vi "Control - Spark.vi"(8 "Control Inputs":T1={"Engine Speed [RPM]"=0.0, "Engine Status"=enum."STALLED", "Load Control \nMode"=enum."Max Speed Governor", "dt(s)"=0.0, "Number of Cylinders"=0, "Engine Displacement [cc]"=0.0, "StoichAFR"=0.0, "Q.LHV Fuel [kJ/kg]"=0.0, "BattV PSU [V]"=0.0, "12V PSU [V]"=0.0, "5V PSU [V]"=0.0, "Pedal Position [%]"=0.0, "Oil Pressure [kPa]"=0.0, "Oil Temp [C]"=0.0, "Oil Level [%]"=0.0, "Engine Coolant Temp (ECT) [C]"=0.0, "Engine Coolant Pressure [kPa]"=0.0, "Rail Pressure [bar]"=0.0, "Fuel Pressure [kPa]"=0.0, "Fuel Temp [C]"=0.0, "Vacuum Pressure [kPa]"=0.0, "Throttle Position [%]"=0.0, "Cam1 Advance [CAD]"=0.0, "Cam2 Advance [CAD]"=0.0, "Cam3 Advance [CAD]"=0.0, "Cam4 Advance [CAD]"=0.0, "CA50 Control Output [CAD]"=[], "CA50 Control Output Valid"=[], "Intake Air Temp (IAT) [C]"=0.0, "Barometric Air Pressure [kPa]"=0.0, "Intake Air Rel. Humidity [%]"=0.0, "Mass Air Flow (MAF) [kg/hr]"=0.0, "Turbo Inlet Air Pressure [kPa]"=0.0, "Turbo Inlet Air Temp [C]"=0.0, "Turbo Outlet Air Pressure [kPa]"=0.0, "Turbo Outlet Air Temp [C]"=0.0, "CAC Outlet Pressure [kPa]"=0.0, "CAC Outlet Temp [C]"=0.0, "Intake Manifold Pressure (MAP) [kPa]"=0.0, "Intake Manifold Temp (MAT) [C]"=0.0, "Exhaust Manifold Pressure [kPa]"=0.0, "Exhaust Manifold Temp [C]"=0.0, "HighP EGR Cooler Outlet Pressure [kPa]"=0.0, "HighP EGR Cooler Outlet Temp [C]"=0.0, "HighP EGR Differential Pressure [kPa]"=0.0, "HighP EGR Valve Position [%]"=0.0, "Turbo Outlet Exhaust Pressure [kPa]"=0.0, "Turbo Outlet Exhaust Temp [C]"=0.0, "VGT Position 1 [%]"=0.0, "VGT Position 2 [%]"=0.0, "Turbo Speed 1 [RPM]"=0.0, "Turbo Speed 2 [RPM]"=0.0, "LowP EGR Differential Pressure [kPa]"=0.0, "LowP EGR Valve Position [%]"=0.0, "UEGO1Lambda"=0.0, "UEGO1_Hot"=FALSE, "UEGO2Lambda"=0.0, "UEGO2_Hot"=FALSE, "Knock Intensity"=[], "Knock"=[]} {"Knock Intensity" format="%.2f"; "CA50 Control Output [CAD]" format="%.2f"; "Exhaust Manifold Temp [C]" format="%#_6f"; "UEGO2Lambda" format="%.2f"; "Intake Manifold Temp (MAT) [C]" format="%#_6f"; "UEGO1Lambda" format="%.2f"}, 10 "EGR Mass [mg/cyc]":sgl, 11 "MEP Desired [bar]":sgl) -> (1 "Spark Timings Desired [DBTDC]":sgl[](array[numeric]), 3 "Spark Dwells Desired [msec]":sgl[](array[numeric]))   [LabVIEW 2015, in "ECS-RT.lvlib"]
uses:
  ECS-RT.lvlib
  Typedefs/Control Inputs/Control Inputs.ctl
  Typedefs/EPT/Engine Status.ctl
  Typedefs/MISC/Load Control Mode.ctl
  ECS-Shared.lvlib
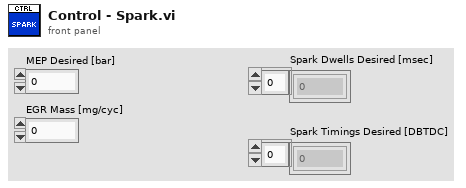
[diagram p1: front panel]
types:
  T1 = typedef "ECS-Shared.lvlib/Control Inputs.ctl" = cluster{"Engine Speed [RPM]":sgl, "Engine Status":T2, "Load Control \nMode":T3, "dt(s)":sgl, "Number of Cylinders":u8, "Engine Displacement [cc]":sgl, "StoichAFR":sgl, "Q.LHV Fuel [kJ/kg]":sgl, "BattV PSU [V]":sgl, "12V PSU [V]":sgl, "5V PSU [V]":sgl, "Pedal Position [%]":sgl, "Oil Pressure [kPa]":sgl, "Oil Temp [C]":sgl, "Oil Level [%]":sgl, "Engine Coolant Temp (ECT) [C]":sgl, "Engine Coolant Pressure [kPa]":sgl, "Rail Pressure [bar]":sgl, "Fuel Pressure [kPa]":sgl, "Fuel Temp [C]":sgl, "Vacuum Pressure [kPa]":sgl, "Throttle Position [%]":sgl, "Cam1 Advance [CAD]":sgl, "Cam2 Advance [CAD]":sgl, "Cam3 Advance [CAD]":sgl, "Cam4 Advance [CAD]":sgl, "CA50 Control Output [CAD]":sgl[], "CA50 Control Output Valid":bool[], "Intake Air Temp (IAT) [C]":sgl, "Barometric Air Pressure [kPa]":sgl, "Intake Air Rel. Humidity [%]":sgl, "Mass Air Flow (MAF) [kg/hr]":sgl, "Turbo Inlet Air Pressure [kPa]":sgl, "Turbo Inlet Air Temp [C]":sgl, "Turbo Outlet Air Pressure [kPa]":sgl, "Turbo Outlet Air Temp [C]":sgl, "CAC Outlet Pressure [kPa]":sgl, "CAC Outlet Temp [C]":sgl, "Intake Manifold Pressure (MAP) [kPa]":sgl, "Intake Manifold Temp (MAT) [C]":sgl, "Exhaust Manifold Pressure [kPa]":sgl, "Exhaust Manifold Temp [C]":sgl, "HighP EGR Cooler Outlet Pressure [kPa]":sgl, "HighP EGR Cooler Outlet Temp [C]":sgl, "HighP EGR Differential Pressure [kPa]":sgl, "HighP EGR Valve Position [%]":sgl, "Turbo Outlet Exhaust Pressure [kPa]":sgl, "Turbo Outlet Exhaust Temp [C]":sgl, "VGT Position 1 [%]":sgl, "VGT Position 2 [%]":sgl, "Turbo Speed 1 [RPM]":sgl, "Turbo Speed 2 [RPM]":sgl, "LowP EGR Differential Pressure [kPa]":sgl, "LowP EGR Valve Position [%]":sgl, "UEGO1Lambda":sgl, "UEGO1_Hot":bool, "UEGO2Lambda":sgl, "UEGO2_Hot":bool, "Knock Intensity":sgl[], "Knock":bool[]}
  T2 = typedef "ECS-Shared.lvlib/Engine Status.ctl" = enum16{"OFF", "STALLED", "CRANKING", "RUNNING", "ACCEL", "DECEL", "SAFE"}
  T3 = typedef "ECS-Shared.lvlib/Load Control Mode.ctl" = enum16{"No Governor", "Min Speed Governor", "Max Speed Governor"}
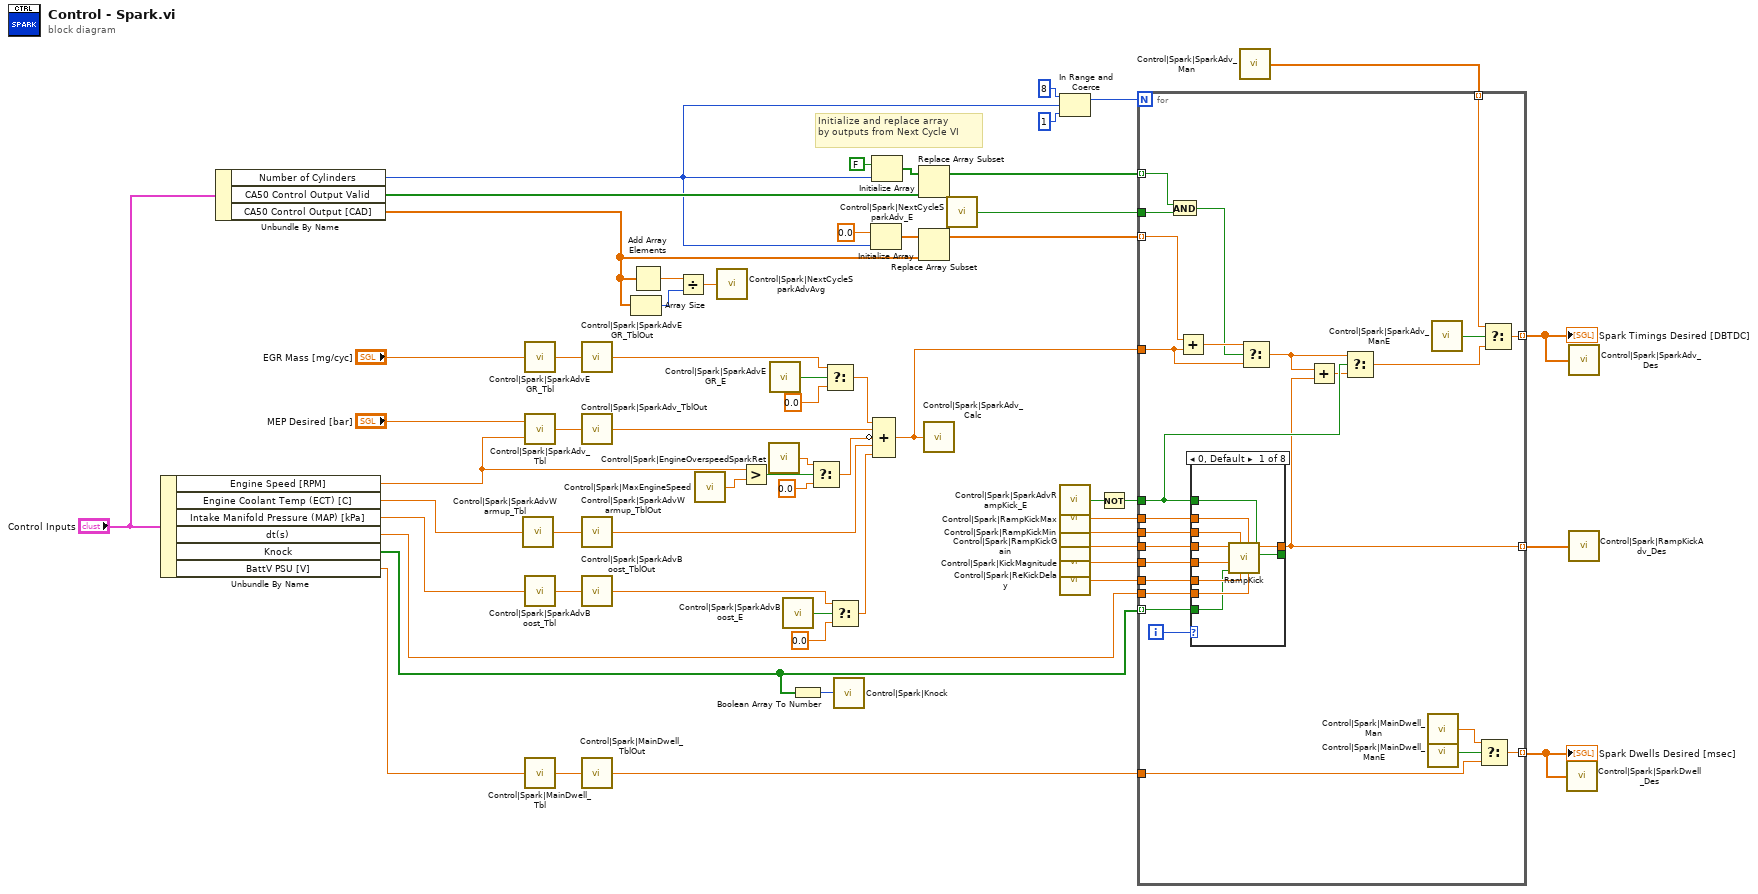
[diagram p0: block diagram]
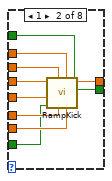
[diagram p2: hidden frame]
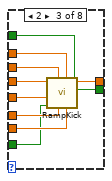
[diagram p3: hidden frame]
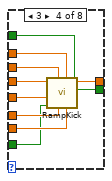
[diagram p4: hidden frame]
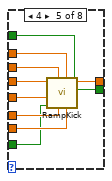
[diagram p5: hidden frame]
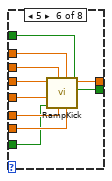
[diagram p6: hidden frame]
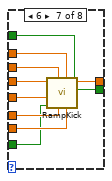
[diagram p7: hidden frame]
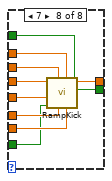
[diagram p8: hidden frame]
diagram:
  # "Initialize and replace array\nby outputs from Next Cycle VI"
  n1 = Unbundle By Name("Control Inputs") -> ("Engine Speed [RPM]"=w26:sgl, "Engine Coolant Temp (ECT) [C]"=w18:sgl, "Intake Manifold Pressure (MAP) [kPa]"=w19:sgl, "dt(s)"=w8:sgl, "Knock"=w7:bool[], "BattV PSU [V]"=w11:sgl)
  n2 = Unbundle By Name("Control Inputs") -> ("Number of Cylinders"=w20:u8, "CA50 Control Output Valid"=w23:bool[], "CA50 Control Output [CAD]"=w22:sgl[])
  n3 = call "Control|Spark|SparkAdvWarmup_Tbl"("X Index"=w18) -> ("Y"=w29:sgl)
  n4 = call "Control|Spark|SparkAdvEGR_Tbl"("X Index"="EGR Mass [mg/cyc]") -> ("Y"=w34:sgl)
  n5 = call "Control|Spark|SparkAdv_Tbl"("Y Index"=w26, "X Index"="MEP Desired [bar]") -> ("Z"=w35:sgl)
  n6 = call "Control|Spark|SparkAdvBoost_Tbl"("X Index"=w19) -> ("Y"=w36:sgl)
  n7 = call "Control|Spark|MainDwell_Tbl"("X Index"=w11) -> ("Y"=w37:sgl)
  n8 = call "Control|Spark|SparkAdvEGR_TblOut"("Value"=w34) -> ()
  n9 = call "Control|Spark|SparkAdv_TblOut"("Value"=w35) -> ()
  n10 = call "Control|Spark|SparkAdvWarmup_TblOut"("Value"=w29) -> ()
  n11 = call "Control|Spark|SparkAdvBoost_TblOut"("Value"=w36) -> ()
  n12 = call "Control|Spark|MainDwell_TblOut"("Value"=w37) -> ()
  n13 = Array Size(array=w22) -> (size(s)=w42:i32)
  n14 = Add Array Elements(numeric array=w22) -> (sum=w43:sgl)
  n15 = Divide(x=w43, y=w42) -> (x/y=w41:sgl)
  n16 = call "Control|Spark|MaxEngineSpeed"() -> ("Value"=w17:sgl)
  n17 = call "Control|Spark|NextCycleSparkAdvAvg"("Value"=w41) -> ()
  n18 = Greater?(x=w26, y=w17) -> (0:w28:bool)
  n19 = call "Control|Spark|EngineOverspeedSparkRet"() -> ("Value"=w25:sgl)
  n20 = call "Control|Spark|SparkAdvEGR_E"() -> ("Value"=w51:bool)
  n21 = call "Control|Spark|SparkAdvBoost_E"() -> ("Value"=w52:bool)
  n22 = Boolean Array To Number(Boolean array=w7) -> (number=w10:u8)
  n23 = Select(t=w25, s=w28, f=sgl 0.0) -> (s? t:f=w27:sgl)
  n24 = Select(t=w34, s=w51, f=sgl 0.0) -> (s? t:f=w48:sgl)
  n25 = Select(t=w36, s=w52, f=sgl 0.0) -> (s? t:f=w30:sgl)
  n26 = call "Control|Spark|Knock"("Value"=w10) -> ()
  n27 = Initialize Array(sgl 0.0, w20) -> (w45:sgl[])
  n28 = Initialize Array(FALSE, w20) -> (w47:bool[])
  n29 = Compound Arithmetic op=ADD(w48, w35, invert w27, w29, w30) -> (w31:sgl)
  n30 = Replace Array Subset(array=w47, new element=w23) -> (w40:bool[])  [unwired: 1 in]
  n31 = Replace Array Subset(array=w45, new element=w22) -> (w39:sgl[])  [unwired: 1 in]
  n32 = call "Control|Spark|SparkAdv_Calc"("Value"=w31) -> ()
  n33 = call "Control|Spark|NextCycleSparkAdv_E"() -> ("Value"=w38:bool)
  n34 = In Range and Coerce(upper limit=u8 8, x=w20, lower limit=u8 1) -> (coerced(x)=w5:u8)  [unwired: 1 out]
  n35 = call "Control|Spark|SparkAdvRampKick_E"() -> ("Value"=w9:bool)
  n36 = call "Control|Spark|RampKickMax"() -> ("Value"=w16:sgl)
  n37 = call "Control|Spark|RampKickMin"() -> ("Value"=w15:sgl)
  n38 = call "Control|Spark|RampKickGain"() -> ("Value"=w14:sgl)
  n39 = call "Control|Spark|KickMagnitude"() -> ("Value"=w13:sgl)
  n40 = call "Control|Spark|ReKickDelay"() -> ("Value"=w12:sgl)
  n41 = Not(x=w9) -> (.not. x?=w6:bool)
  n42 = call "Control|Spark|SparkAdv_Man"() -> ("Value"=w1:sgl[])
  n43 = for {
    N: w5 -> [_]
    tunnel: w31 -> [w74]
    tunnel: w37 -> [w78]
    tunnel: [w77] -> w32 mode=indexing
    tunnel: [w76] -> w33 mode=indexing
    tunnel: w40 -> [w71] mode=indexing
    tunnel: w39 -> [w73] mode=indexing
    tunnel: w38 -> [w70]
    tunnel: w16 -> [w67]
    tunnel: w15 -> [w66]
    tunnel: w14 -> [w65]
    tunnel: w13 -> [w64]
    tunnel: w12 -> [w63]
    tunnel: w8 -> [w62]
    tunnel: w7 -> [w61] mode=indexing
    tunnel: w6 -> [w59]
    tunnel: [w56] -> w2 mode=indexing
    tunnel: w1 -> [w55] mode=indexing
    i -> [w68]
    n44 = And(x=w71, y=w70) -> (x .and. y?=w69:bool)
    n45 = Add(x=w73, y=w74) -> (x+y=w75:sgl)
    n46 = case shown="0, Default" w68 {
      tunnel: w66 -> [w90 w100 w110 w120 w130 w140 w150 w160]
      tunnel: w67 -> [w89 w99 w109 w119 w129 w139 w149 w159]
      tunnel: w65 -> [w88 w98 w108 w118 w128 w138 w148 w158]
      tunnel: w64 -> [w87 w97 w107 w117 w127 w137 w147 w157]
      tunnel: w63 -> [w86 w96 w106 w116 w126 w136 w146 w156]
      tunnel: w62 -> [w85 w95 w105 w115 w125 w135 w145 w155]
      tunnel: w61 -> [w84 w94 w104 w114 w124 w134 w144 w154]
      tunnel: [w83 w93 w103 w113 w123 w133 w143 w153] -> w56
      tunnel: [w82 w92 w102 w112 w122 w132 w142 w152] -> _
      tunnel: w59 -> [w81 w91 w101 w111 w121 w131 w141 w151]
      frame 0, Default {
        n47 = call "RampKick.vi"("Init (F)"=w81, "dt [s]"=w85, "Output Max [unit]"=w89, "Re-Kick Delay [s]"=w86, "Output Min [unit]"=w90, "Kick?"=w84, "Kick Magnitude [unit]"=w87, "Gain [unit/s]"=w88) -> ("Kicked"=w82:bool, "Ramp/Kick Output"=w83:sgl)  [unwired: 2 in]
      }
      frame 1 {
        n48 = call "RampKick.vi"("Init (F)"=w91, "dt [s]"=w95, "Output Max [unit]"=w99, "Re-Kick Delay [s]"=w96, "Output Min [unit]"=w100, "Kick?"=w94, "Kick Magnitude [unit]"=w97, "Gain [unit/s]"=w98) -> ("Kicked"=w92:bool, "Ramp/Kick Output"=w93:sgl)  [unwired: 2 in]
      }
      frame 2 {
        n49 = call "RampKick.vi"("Init (F)"=w101, "dt [s]"=w105, "Output Max [unit]"=w109, "Re-Kick Delay [s]"=w106, "Output Min [unit]"=w110, "Kick?"=w104, "Kick Magnitude [unit]"=w107, "Gain [unit/s]"=w108) -> ("Kicked"=w102:bool, "Ramp/Kick Output"=w103:sgl)  [unwired: 2 in]
      }
      frame 3 {
        n50 = call "RampKick.vi"("Init (F)"=w111, "dt [s]"=w115, "Output Max [unit]"=w119, "Re-Kick Delay [s]"=w116, "Output Min [unit]"=w120, "Kick?"=w114, "Kick Magnitude [unit]"=w117, "Gain [unit/s]"=w118) -> ("Kicked"=w112:bool, "Ramp/Kick Output"=w113:sgl)  [unwired: 2 in]
      }
      frame 4 {
        n51 = call "RampKick.vi"("Init (F)"=w121, "dt [s]"=w125, "Output Max [unit]"=w129, "Re-Kick Delay [s]"=w126, "Output Min [unit]"=w130, "Kick?"=w124, "Kick Magnitude [unit]"=w127, "Gain [unit/s]"=w128) -> ("Kicked"=w122:bool, "Ramp/Kick Output"=w123:sgl)  [unwired: 2 in]
      }
      frame 5 {
        n52 = call "RampKick.vi"("Init (F)"=w131, "dt [s]"=w135, "Output Max [unit]"=w139, "Re-Kick Delay [s]"=w136, "Output Min [unit]"=w140, "Kick?"=w134, "Kick Magnitude [unit]"=w137, "Gain [unit/s]"=w138) -> ("Kicked"=w132:bool, "Ramp/Kick Output"=w133:sgl)  [unwired: 2 in]
      }
      frame 6 {
        n53 = call "RampKick.vi"("Init (F)"=w141, "dt [s]"=w145, "Output Max [unit]"=w149, "Re-Kick Delay [s]"=w146, "Output Min [unit]"=w150, "Kick?"=w144, "Kick Magnitude [unit]"=w147, "Gain [unit/s]"=w148) -> ("Kicked"=w142:bool, "Ramp/Kick Output"=w143:sgl)  [unwired: 2 in]
      }
      frame 7 {
        n54 = call "RampKick.vi"("Init (F)"=w151, "dt [s]"=w155, "Output Max [unit]"=w159, "Re-Kick Delay [s]"=w156, "Output Min [unit]"=w160, "Kick?"=w154, "Kick Magnitude [unit]"=w157, "Gain [unit/s]"=w158) -> ("Kicked"=w152:bool, "Ramp/Kick Output"=w153:sgl)  [unwired: 2 in]
      }
    }
    n55 = Select(t=w75, s=w69, f=w74) -> (s? t:f=w57:sgl)
    n56 = Add(x=w57, y=w56) -> (x+y=w58:sgl)
    n57 = Select(t=w57, s=w59, f=w58) -> (s? t:f=w60:sgl)
    n58 = call "Control|Spark|MainDwell_Man"() -> ("Value"=w72:sgl)
    n59 = call "Control|Spark|MainDwell_ManE"() -> ("Value"=w79:bool)
    n60 = call "Control|Spark|SparkAdv_ManE"() -> ("Value"=w80:bool)
    n61 = Select(t=w72, s=w79, f=w78) -> (s? t:f=w77:sgl)
    n62 = Select(t=w55, s=w80, f=w60) -> (s? t:f=w76:sgl)
  }
  "Spark Timings Desired [DBTDC]" <- w33
  "Spark Dwells Desired [msec]" <- w32
  n63 = call "Control|Spark|SparkDwell_Des"("Value"=w32) -> ()
  n64 = call "Control|Spark|SparkAdv_Des"("Value"=w33) -> ()
  n65 = call "Control|Spark|RampKickAdv_Des"("Value"=w2) -> ()
